vi "Part 2.vi"(11 "Input":string) -> (3 "Output":i64)   [LabVIEW 2021]
uses:
  <userlib>/_OpenG.lib/string/string.llb/Convert EOLs (String)__ogtk.vi
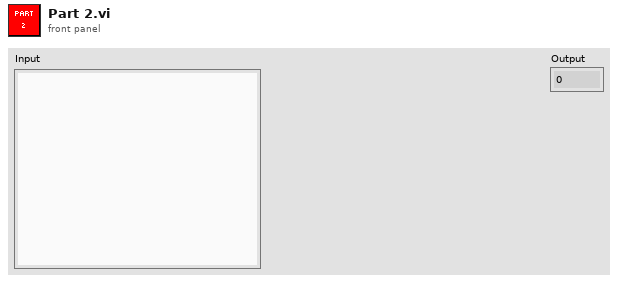
[diagram p1: front panel]
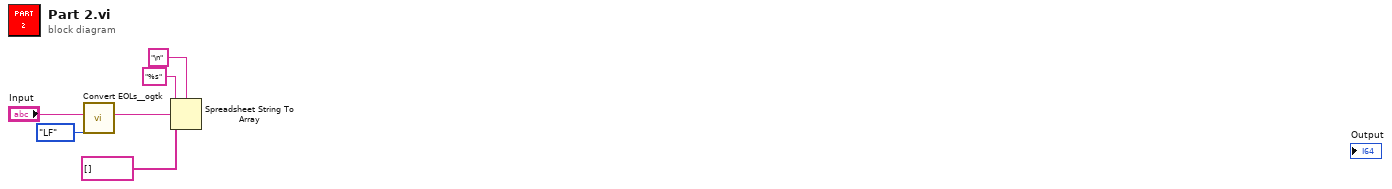
[diagram p0: block diagram]
diagram:
  n1 = call-poly <userlib>:"Convert EOLs__ogtk.vi"("Convert to:"=enum16{"CR", "LF", "CRLF"}."LF", "String in"="Input") -> ("String out"=w2:string)  [unwired: 9 in]
  n2 = Spreadsheet String To Array(delimiter (Tab)="\n", format string="%s", spreadsheet string=w2, array type (2D Dbl)=string[] []) -> ()  [unwired: 1 out]
